vi "Trigger.vi"(8 "Error In":errorcluster, 11 "reference in":refnum<class "ByRef1.lvclass">) -> (0 "Error Out":errorcluster, 3 "reference out":refnum<class "ByRef1.lvclass">)   [LabVIEW 2020, in "ByRef1.lvclass"]
doc: "This method gets called every time the trigger elaps"
uses:
  ByRef1.lvclass
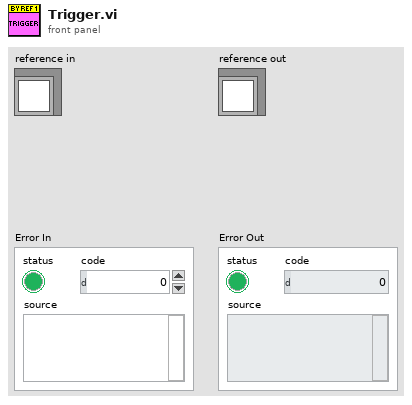
[diagram p1: front panel]
types:
  T1 = typedef "ByRef1.lvclass/ObjectAttributes.ctl" = cluster{"Triggers":i32}
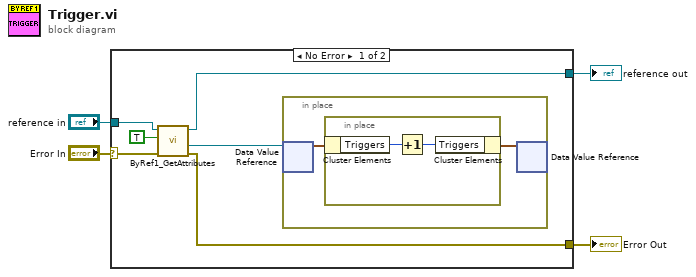
[diagram p0: block diagram]
diagram:
  n1 = case shown="No Error" "Error In" {
    selector: "Error In" -> [w10 w16]
    tunnel: [w9 w16] -> w3
    tunnel: [w7 w15] -> w1
    tunnel: "reference in" -> [w8 w15]
    frame No Error {
      n2 = call "ByRef1_GetAttributes.vi"("error in (no error)"=w10, "OnlyGetDvrReference(False)"=TRUE, "reference in"=w8) -> ("error out"=w9:errorcluster, "DataRef"=w5:refnum<data-value>, "reference out"=w7:refnum<class "ByRef1.lvclass">)  [unwired: 5 in, 1 out]
      n3 = in-place {
        n4 = in-place-dvr #1(w5) -> (w12:T1)  [unwired: 1 out]
        n5 = in-place {
          n6 = in-place-cluster #2(w12) -> ("Triggers"=w14:i32)
          n7 = Increment(x=w14) -> (x+1=w13:i32)
          n8 = in-place-cluster #2("Triggers"=w13) -> (w11:T1)
        }
        n9 = in-place-dvr #1(w11) -> ()  [unwired: 2 out]
      }
    }
    frame Error {
    }
  }
  "Error Out" <- w3
  "reference out" <- w1
